vi "SWITCH Initialize Hardware References.vi"(8 "error in (no error)":errorcluster, 11 "Hardware Resources in":T1={"Tango HW"={"VISA resource"="", "Baud Rate (115200)"=2, "lAnInterfaceType"=0, "bAShowProt"=15}, "Writer Queue"=refnum, "Status"=FALSE, "Abs Position"=[], "Axis Velocity"={"dX"=0.0, "dY"=0.0, "dZ"=0.0, "dA"=0.0}, "acceleration "=0.0, "Z direction"=enum."Up", "Position Mode"="", "plLSID"=0}) -> (0 "error out":errorcluster, 3 "Hardware Resources out":T1={"Tango HW"={"VISA resource"="", "Baud Rate (115200)"=2, "lAnInterfaceType"=0, "bAShowProt"=15}, "Writer Queue"=refnum, "Status"=FALSE, "Abs Position"=[], "Axis Velocity"={"dX"=0.0, "dY"=0.0, "dZ"=0.0, "dA"=0.0}, "acceleration "=0.0, "Z direction"=enum."Up", "Position Mode"="", "plLSID"=0})   [LabVIEW 2020, in "MOTOR.lvlib"]
doc: "Initialize the hardware references."
uses:
  MOTOR.lvlib
  PS Hardware Configuration.ctl
  support/Message Queue/Message Cluster.ctl
  support/PCT FGV CMD.ctl
  <instrlib>/Tango_DLL/Tango_DLL.lvlib
  support/Message Queue/Message Queue.lvlib
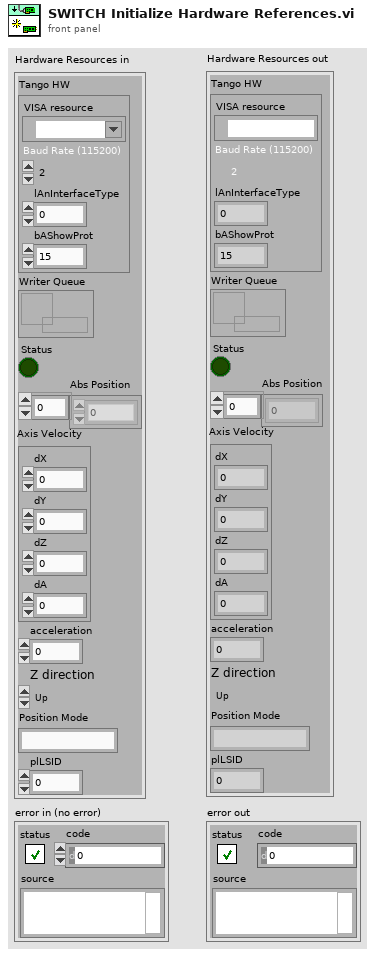
[diagram p1: front panel]
types:
  T1 = typedef "MOTOR.lvlib/PS Hardware Configuration.ctl" = cluster{"Tango HW":cluster{"VISA resource":refnum<visa-resource-name>, "Baud Rate (115200)":i32, "lAnInterfaceType":i32, "bAShowProt":i32}, "Writer Queue":refnum<queue>, "Status":bool, "Abs Position":i32[], "Axis Velocity":cluster{"dX":dbl, "dY":dbl, "dZ":dbl, "dA":dbl}, "acceleration ":dbl, "Z direction":enum16{"Up", "Down"}, "Position Mode":string, "plLSID":i32}
  T2 = typedef "PCT FGV CMD.ctl" = enum16{"INIT", "GET", "SET"}
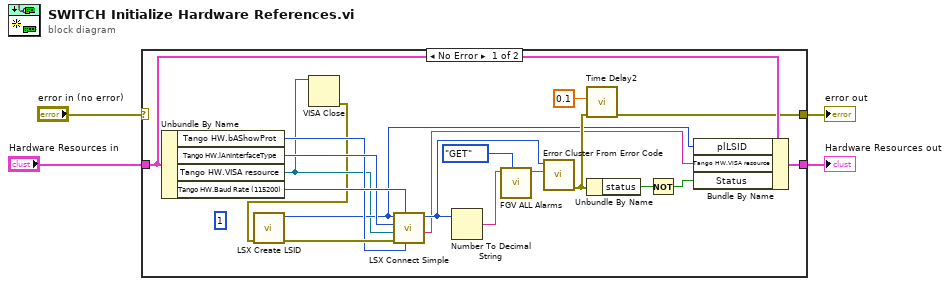
[diagram p0: block diagram]
diagram:
  n1 = case shown="No Error" "error in (no error)" {
    selector: "error in (no error)" -> [_ w24]
    tunnel: [w19 w24] -> w3
    tunnel: "Hardware Resources in" -> [w22 w25]
    tunnel: [w23 w25] -> w1
    frame No Error {
      (unwired) 1 ("lAnInterfaceType")
      n2 = Unbundle By Name(w22) -> ("Tango HW.bAShowProt"=w9:i32, "Tango HW.lAnInterfaceType"=w10:i32, "Tango HW.VISA resource"=w6:refnum<visa-resource-name>, "Tango HW.Baud Rate (115200)"=w11:i32)
      n3 = VISA Close(VISA resource name=w6) -> (error out=w5:errorcluster)  [unwired: 1 in]
      n4 = call <instrlib>:"LSX Create LSID.vi"("error in (no error)"=w5) -> ("error out"=w13:errorcluster, "plLSID out"=w7:i32)  [unwired: 8 in, 1 out]
      n5 = call <instrlib>:"LSX Connect Simple.vi"("bAShowProt"=w9, "lABaudRate"=w11, "error in (no error)"=w13, "pcAComName"=w6, "lAnInterfaceType"=w10, "lLSID"=w7) -> ("pcAComName out"=w8:string, "function return"=w12:i32)  [unwired: 3 in, 1 out]
      n6 = Number To Decimal String(number=w12) -> (decimal integer string=w15:string)  [unwired: 1 in]
      n7 = call "FGV ALL Alarms.vi"("CMD"=PCT_FGV_CMD."GET", "name"=w15) -> ("Alarm MSG out"=w14:string)  [unwired: 8 in, 1 out]
      n8 = call <vilib>:"Error Cluster From Error Code.vi"("error message (\"\")"=w14, "error code (0)"=w12) -> ("error out"=w17:errorcluster)  [unwired: 7 in]
      n9 = call "Time Delay2"("error in (no error)"=w17, "Delay Time (s)"=0.1) -> ("error out"=w19:errorcluster)  [unwired: 9 in]
      n10 = Unbundle By Name(w17) -> ("status"=w20:bool)
      n11 = Not(x=w20) -> (.not. x?=w21:bool)
      n12 = Bundle By Name(cluster=w22, "plLSID"=w7, "Tango HW.VISA resource"=w8, "Status"=w21) -> (w23:T1)
    }
    frame Error {
    }
  }
  "Hardware Resources out" <- w1
  "error out" <- w3
